vi "Ej 10 Inicializar Variables.vi"() -> ()   [LabVIEW 2021]
panel:
  out "Indicador Contraseña":string
  out "Indicador Nombre":string
  in  "Contraseña":string
  in  "Nombre":string
  in  "stop":bool
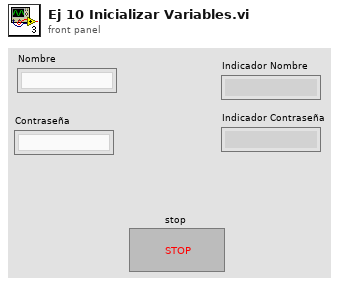
[diagram p1: front panel]
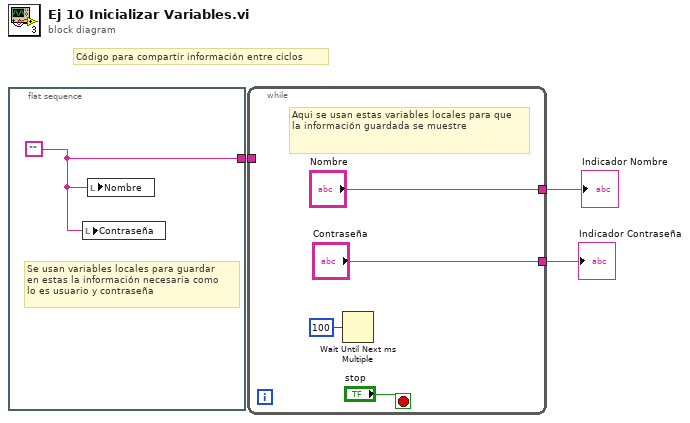
[diagram p0: block diagram]
diagram:
  # "Código para compartir información entre ciclos"
  n1 = flat-sequence {
    tunnel: [w4] -> w1
    frame #0 {
      w4 = ""
      # "Se usan variables locales para guardar\nen estas la información necesaria como \nlo es usuario y contraseña"
      n2 = local write "Contraseña"(w4) -> ()
      n3 = local write "Nombre"(w4) -> ()
    }
  }
  n4 = while {
    tunnel: ["Nombre"] -> w3
    tunnel: ["Contraseña"] -> w2
    tunnel: w1 -> [_]
    stop <- "stop" stop-if-true
    # "Aqui se usan estas variables locales para que \nla información guardada se muestre"
    n5 = Wait Until Next ms Multiple(millisecond multiple=u32 100) -> ()  [unwired: 1 out]
  }
  "Indicador Nombre" <- w3
  "Indicador Contraseña" <- w2
